vi "Main.vi"(7 "Action":T1=enum."Close", 8 "Error In":errorcluster, 11 "Data In":variant) -> (0 "Error Out":errorcluster, 3 "Data Out":variant)   [LabVIEW 2018, in "Receipt Parsing.lvlib"]
doc: "Action Engine for the module. This private VI is wrapped for the API."
uses:
  Receipt Parsing.lvlib
  Action.ctl
  <vilib>/vision/Image Controls.llb/IMAQ Image.ctl
  Provisional Parsed Values--cluster.ctl
  ReceiptItemInfo.ctl
  <vilib>/vision/OCR.llb/IMAQ OCR Session.ctl
  Section Info--cluster.ctl
  <vilib>/Utility/error.llb/Error Cluster From Error Code.vi
  <vilib>/ErrorRing/Error Ring.xnode
  <vilib>/vision/NI_Vision_Development_Module.lvlib
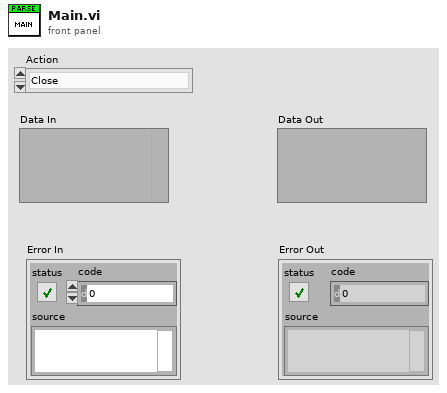
[diagram p1: front panel]
types:
  T1 = typedef "Receipt Parsing.lvlib/Action.ctl" = enum16{"Init", "Read Image Text", "Text Get Sections", "Sections Get Data", "Close"}
  T2 = typedef "ROI Descriptor" = cluster{"Global Rectangle":i32[], "Contours":cluster{"ID":enum32{"External", "Internal"}, "Type":u32, "Coordinates":i32[]}[]}
  T3 = typedef "IMAQ Image.ctl" = refnum<image>
  T4 = cluster{"Receipt Lines":string[], "Rows Where Whitespace Starts":i32[]}
  T5 = typedef "IMAQ OCR Session.ctl" = refnum<k1>
  T6 = typedef "Receipt Parsing.lvlib/Section Info--cluster.ctl" = cluster{"Text Lines":string[], "Text":string, "Section Start Row (pix)":i32, "Section End Row (pix)":i32}
  T7 = typedef "Receipt Parsing.lvlib/Provisional Parsed Values--cluster.ctl" = cluster{"Location":string, "Line Items ":T8[], "TotalPrice":dbl, "DateTime":timestamp}
  T8 = typedef "Receipt Parsing.lvlib/ReceiptItemInfo.ctl" = cluster{"Unit":string, "TaxStatus":string, "PrintedName":string, "ItemName":string, "NumberOfUnits":dbl, "PriceIncDiscount (£)":dbl, "Discount(£)":dbl, "Error?":bool}
  T9 = cluster{"IMAQ OCR Session":T5, "Header Info":T6, "Main Body Info":T6, "Footer Info":T6, "Provisional Parsed Values":T7}
  T10 = typedef "Receipt Parsing.lvlib/Line Number.ctl" = cluster{"End of Header":i32, "Start of Main":i32, "Start of Footer":i32}
  T11 = cluster{"Header Info":T6, "Main Body Info":T6, "Footer Info":T6}
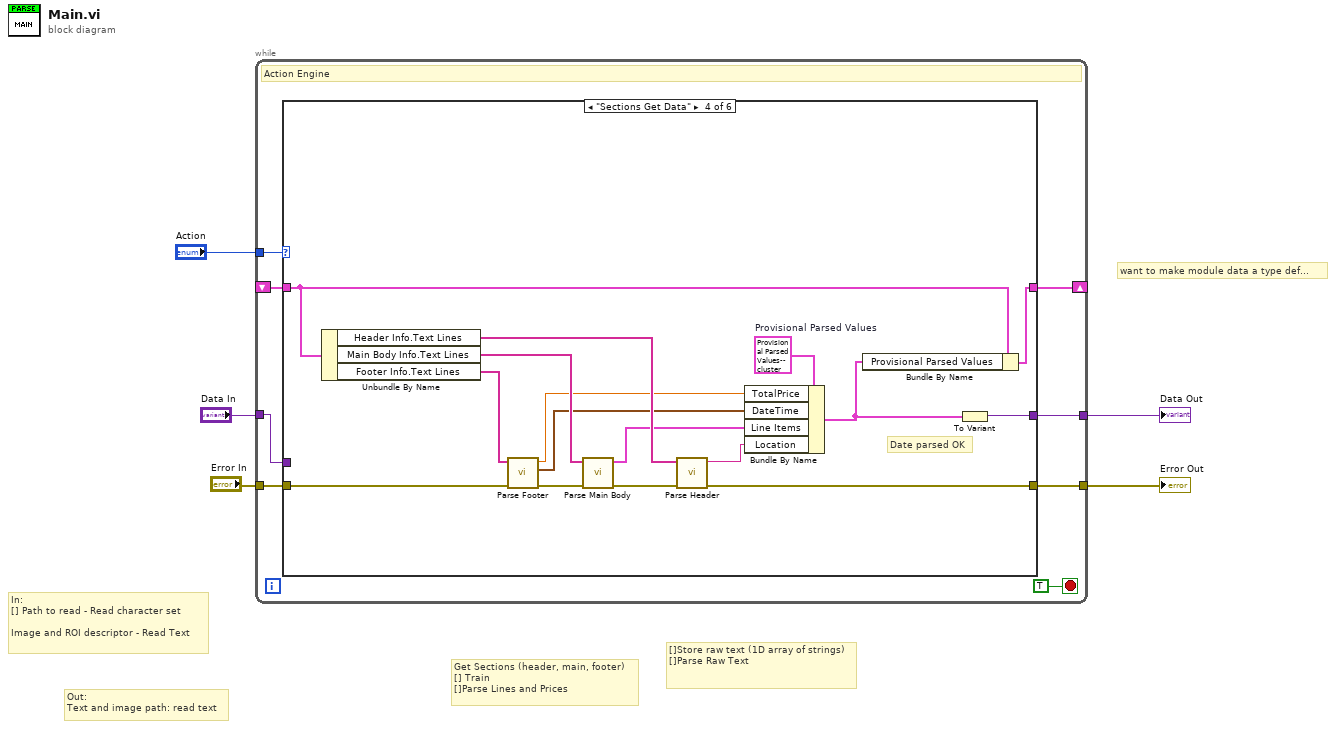
[diagram p0: block diagram]
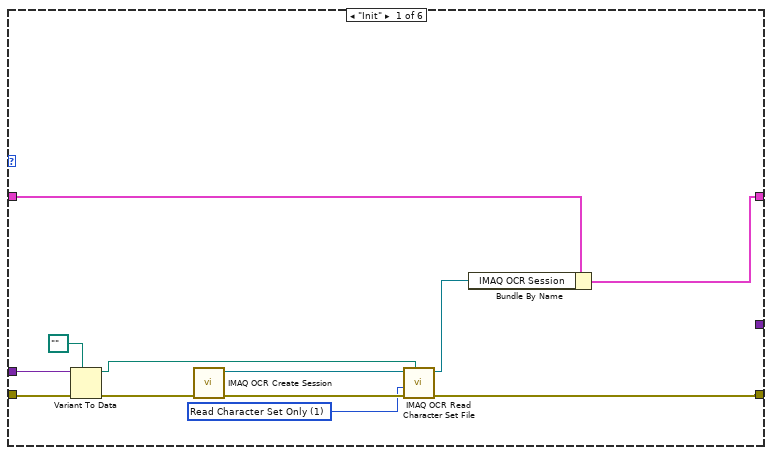
[diagram p2: hidden frame]
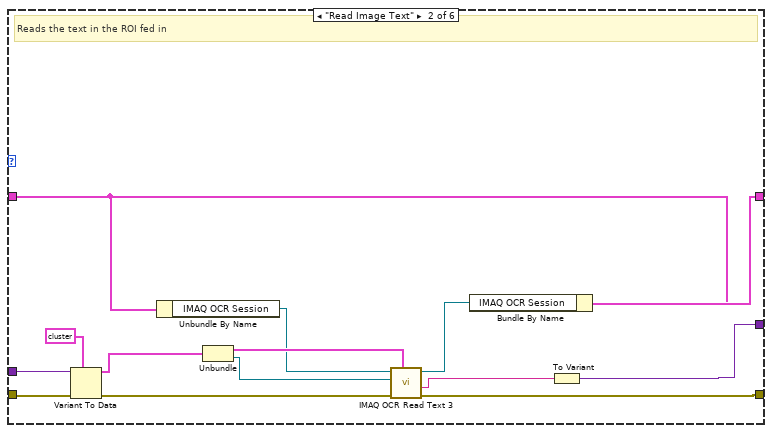
[diagram p3: hidden frame]
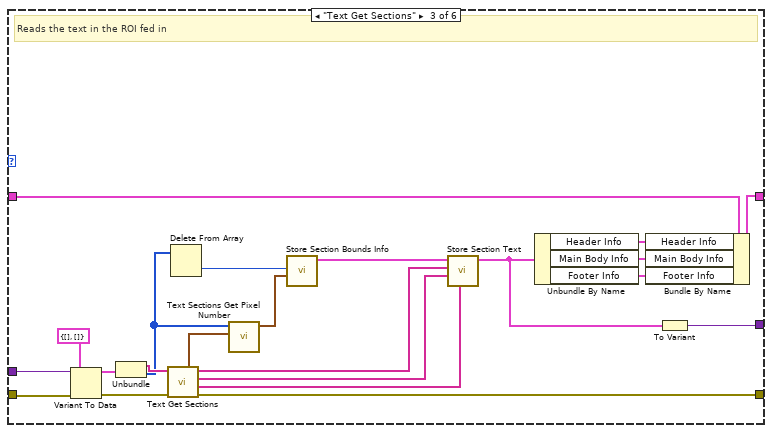
[diagram p4: hidden frame]
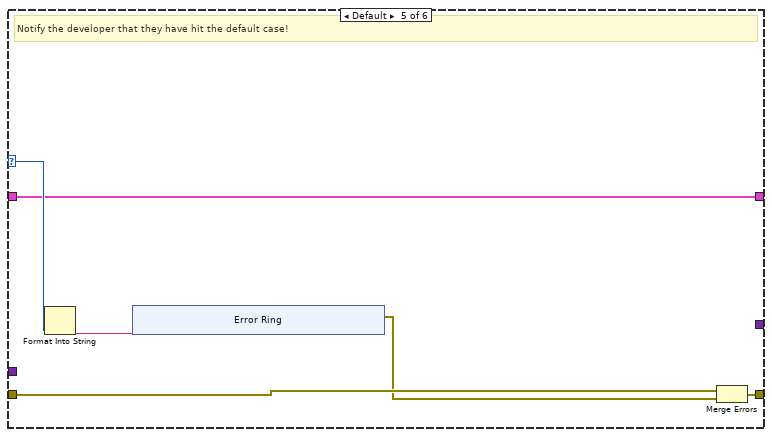
[diagram p5: hidden frame]
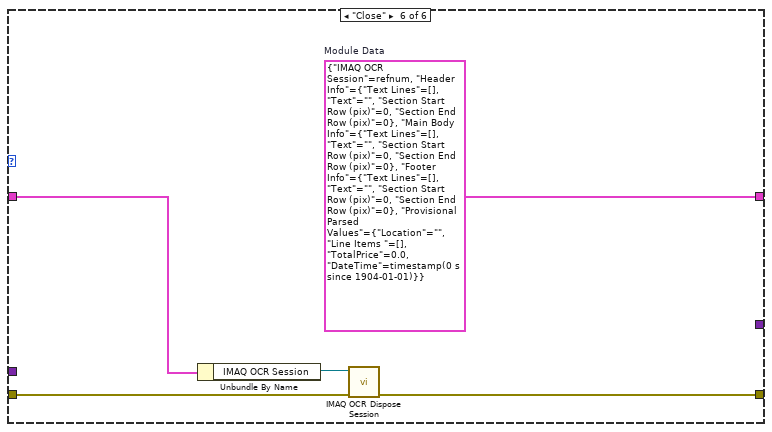
[diagram p6: hidden frame]
diagram:
  # "want to make module data a type def..."
  # "[]Store raw text (1D array of strings)\n[]Parse Raw Text"
  # "Get Sections (header, main, footer)\n[] Train\n[]Parse Lines and Prices"
  # "Out:\nText and image path: read text"
  # "In:\n[] Path to read - Read character set\n\nImage and ROI descriptor - Read Text"
  n1 = while {
    tunnel: "Error In" -> [w11]
    tunnel: [w12] -> w4
    tunnel: "Action" -> [w10]
    shift-right: [w9] -> _
    shift-left: _ -> [w8]
    tunnel: "Data In" -> [w7]
    tunnel: [w6] -> w1
    stop <- TRUE stop-if-true
    # "Action Engine"
    n2 = case shown="\"Sections Get Data\"" w10 {
      selector: w10 -> [_ _ _ _ w79 _]
      tunnel: [w22 w35 w59 w74 w83 w95] -> w12
      tunnel: w11 -> [w17 w38 w61 w71 w82 w94]
      tunnel: [w19 w39 w42 w64 w78 w91] -> w9
      tunnel: w8 -> [w21 w30 w46 w65 w78 w92]
      tunnel: w7 -> [w15 w37 w60 _ _ _]
      tunnel: [_ w26 w41 w63 _ _] -> w6
      frame "Init" {
        w23 = 1 items=["Read All", "Read Character Set Only", "Read Properties Only"] ("Read Options")
        n3 = Variant To Data(error in=w17, type=path "" ("File Path"), Variant=w15) -> (data=w14:path, error out=w18:errorcluster)
        n4 = call "IMAQ OCR Create Session"("error in (no error)"=w18) -> ("error out"=w25:errorcluster, "IMAQ OCR Session"=w24:T5)  [unwired: 9 in]
        n5 = call "IMAQ OCR Read Character Set File"("File Path"=w14, "error in (no error)"=w25, "Read Options"=w23, "IMAQ OCR Session"=w24) -> ("error out"=w22:errorcluster, "IMAQ OCR Session (dup)"=w20:T5)  [unwired: 5 in, 1 out]
        n6 = Bundle By Name(cluster=w21, "IMAQ OCR Session"=w20) -> (w19:T9)
      }
      frame "Read Image Text" {
        # "Reads the text in the ROI fed in"
        n7 = Variant To Data(error in=w38, type=cluster{"ROI Descriptor":T2, "Image Out":T3} {"ROI Descriptor"={"Global Rectangle"=[], "Contours"=[]}, "Image Out"=refnum} ("output cluster"), Variant=w37) -> (data=w33:cluster{"ROI Descriptor":T2, "Image Out":T3}, error out=w36:errorcluster)
        n8 = Unbundle By Name(w30) -> ("IMAQ OCR Session"=w29:T5)
        n9 = Unbundle(w33) -> ("ROI Descriptor"=w31:T2, "Image Out"=w32:T3)
        n10 = call "IMAQ OCR Read Text 3"("ROI Descriptor"=w31, "error in (no error)"=w36, "Image"=w32, "IMAQ OCR Session"=w29) -> ("error out"=w35:errorcluster, "Read String"=w27:string, "IMAQ OCR Session (dup)"=w28:T5)  [unwired: 2 in, 3 out]
        n11 = Bundle By Name(cluster=w30, "IMAQ OCR Session"=w28) -> (w39:T9)
        n12 = To Variant(anything=w27) -> (Variant=w26:variant)
      }
      frame "Text Get Sections" {
        # "Reads the text in the ROI fed in"
        n13 = Variant To Data(error in=w61, type=T4 {"Receipt Lines"=[], "Rows Where Whitespace Starts"=[]} ("cluster"), Variant=w60) -> (data=w50:T4, error out=w58:errorcluster)
        n14 = Unbundle(w50) -> ("Receipt Lines"=w49:string[], "Rows Where Whitespace Starts"=w47:i32[])
        n15 = call "Text Get Sections.vi"("Error In"=w58, "Receipt Lines"=w49) -> ("Error Out"=w59:errorcluster, "Footer"=w54:string[], "Main Body"=w55:string[], "End of Header"=w56:string[], "Line Numbers"=w53:T10)  [unwired: 5 in]
        n16 = Delete From Array(array=w47) -> (deleted portion=w48:i32)  [unwired: 2 in, 1 out]
        n17 = call "Text Sections Get Pixel Number.vi"("Line Numbers"=w53, "Rows where whitespace starts"=w47) -> ("Line Pixel Value (Vertical)"=w52:T10)  [unwired: 5 in, 4 out]
        n18 = call "Store Section Bounds Info.vi"("Line Numbers"=w52, "Last row"=w48) -> ("Section Data out"=w57:T11)  [unwired: 9 in]
        n19 = call "Store Section Text.vi"("Footer"=w54, "Main Body"=w55, "End of Header"=w56, "Section Data in"=w57) -> ("Section Data out"=w40:T11)  [unwired: 7 in]
        n20 = Unbundle By Name(w40) -> ("Header Info"=w45:T6, "Main Body Info"=w44:T6, "Footer Info"=w43:T6)
        n21 = Bundle By Name(cluster=w46, "Header Info"=w45, "Main Body Info"=w44, "Footer Info"=w43) -> (w42:T9)
        n22 = To Variant(anything=w40) -> (Variant=w41:variant)
      }
      frame "Sections Get Data" {
        w70 = T7 {"Location"="", "Line Items "=[], "TotalPrice"=0.0, "DateTime"=timestamp(0 s since 1904-01-01)}  # Provisional Parsed Values
        # "Date parsed OK"
        n23 = Unbundle By Name(w65) -> ("Header Info.Text Lines"=w77:string[], "Main Body Info.Text Lines"=w76:string[], "Footer Info.Text Lines"=w75:string[])
        n24 = call "Parse Footer.vi"("error in"=w71, "Footer"=w75) -> ("error out"=w72:errorcluster, "DateTime"=w66:timestamp, "TotalPrice"=w67:dbl)  [unwired: 7 in]
        n25 = call "Parse Main Body.vi"("Error In"=w72, "Main Body"=w76) -> ("Error Out"=w73:errorcluster, "Provisional Line Items"=w68:T8[])  [unwired: 8 in]
        n26 = call "Parse Header.vi"("error in (no error)"=w73, "Header"=w77) -> ("error out"=w74:errorcluster, "Location"=w69:string)  [unwired: 8 in]
        n27 = Bundle By Name(cluster=w70, "TotalPrice"=w67, "DateTime"=w66, "Line Items"=w68, "Location"=w69) -> (w62:T7)
        n28 = Bundle By Name(cluster=w65, "Provisional Parsed Values"=w62) -> (w64:T9)
        n29 = To Variant(anything=w62) -> (Variant=w63:variant)
      }
      frame Default {
        # "Notify the developer that they have hit the default case!"
        n30 = Format Into String(w79) -> (resulting string=w80:string)  [unwired: 3 in, 1 out]
        n31 = xnode "Error Ring"("parameter 0"=w80) -> ("error out"=w81:errorcluster)
        n32 = Merge Errors(w82, w81) -> (w83:errorcluster)
      }
      frame "Close" {
        w91 = T9 {"IMAQ OCR Session"=refnum, "Header Info"={"Text Lines"=[], "Text"="", "Section Start Row (pix)"=0, "Section End Row (pix)"=0}, "Main Body Info"={"Text Lines"=[], "Text"="", "Section Start Row (pix)"=0, "Section End Row (pix)"=0}, "Footer Info"={"Text Lines"=[], "Text"="", "Section Start Row (pix)"=0, "Section End Row (pix)"=0}, "Provisional Parsed Values"={"Location"="", "Line Items "=[], "TotalPrice"=0.0, "DateTime"=timestamp(0 s since 1904-01-01)}}  # Module Data
        n33 = Unbundle By Name(w92) -> ("IMAQ OCR Session"=w93:T5)
        n34 = call "IMAQ OCR Dispose Session"("error in (no error)"=w94, "IMAQ OCR Session"=w93) -> ("error out"=w95:errorcluster)  [unwired: 9 in]
      }
    }
  }
  "Error Out" <- w4
  "Data Out" <- w1
